vi "Configure Power Analysis.vi"   [LabVIEW 2015, in "Agilent 2000 3000 X-Series.lvlib"]
doc: "Configures power analysis."
uses:
  <instrlib>/Agilent 2000 3000 X-Series/Agilent 2000 3000 X-Series.lvlib
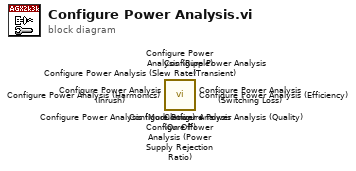
[diagram p0: block diagram]
diagram:
  n1 = call <instrlib>:"Configure Power Analysis (On Off).vi"() -> ()  [unwired: 10 in, 2 out]
  n2 = call <instrlib>:"Configure Power Analysis (Transient).vi"() -> ()  [unwired: 10 in, 2 out]
  n3 = call <instrlib>:"Configure Power Analysis (Inrush).vi"() -> ()  [unwired: 10 in, 2 out]
  n4 = call <instrlib>:"Configure Power Analysis (Switching Loss).vi"() -> ()  [unwired: 10 in, 2 out]
  n5 = call <instrlib>:"Configure Power Analysis (Slew Rate).vi"() -> ()  [unwired: 10 in, 2 out]
  n6 = call <instrlib>:"Configure Power Analysis (Ripple).vi"() -> ()  [unwired: 10 in, 2 out]
  n7 = call <instrlib>:"Configure Power Analysis (Quality).vi"() -> ()  [unwired: 10 in, 2 out]
  n8 = call <instrlib>:"Configure Power Analysis (Power Supply Rejection Ratio).vi"() -> ()  [unwired: 10 in, 2 out]
  n9 = call <instrlib>:"Configure Power Analysis (Modulation).vi"() -> ()  [unwired: 10 in, 2 out]
  n10 = call <instrlib>:"Configure Power Analysis (Harmonics).vi"() -> ()  [unwired: 10 in, 2 out]
  n11 = call <instrlib>:"Configure Power Analysis (Efficiency).vi"() -> ()  [unwired: 10 in, 2 out]
